vi "VI Tree.vi"   [LabVIEW 2013, in "Fluke 2625A.lvlib"]
doc: "This is the instrument driver for the <INSTRUMENT NAME>. The VI Tree displays all the user-callable VIs of the instrument driver in an organized table."
uses:
  <instrlib>/Fluke 2625A/Fluke 2625A.lvlib
panel:
  # "(c) 2007 <Enter Company Name Here>.  ALL RIGHTS RESERVED."
  # "SEE DIAGRAM\nFOR VI TREE."
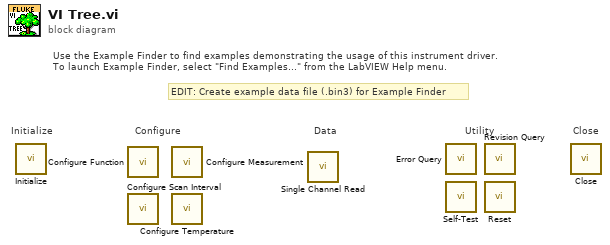
[diagram p0: block diagram]
diagram:
  # "EDIT: Create example data file (.bin3) for Example Finder"
  # "Use the Example Finder to find examples demonstrating the usage of this instrument driver.\nTo launch Example Finder, select \"Find Examples...\" from the LabVIEW Help menu."
  # "Configure"
  # "Utility"
  # "Data"
  # "Close"
  # "Initialize"
  n1 = call <instrlib>:"Initialize.vi"() -> ()  [unwired: 9 in, 3 out]
  n2 = call <instrlib>:"Configure Function.vi"() -> ()  [unwired: 12 in, 4 out]
  n3 = call <instrlib>:"Configure Scan Interval.vi"() -> ()  [unwired: 10 in, 2 out]
  n4 = call <instrlib>:"Configure Measurement.vi"() -> ()  [unwired: 10 in, 2 out]
  n5 = call <instrlib>:"Configure Temperature.vi"() -> ()  [unwired: 9 in, 3 out]
  n6 = call <instrlib>:"Single Channel Read.vi"() -> ()  [unwired: 7 in, 5 out]
  n7 = call <instrlib>:"Error Query.vi"() -> ()  [unwired: 8 in, 4 out]
  n8 = call <instrlib>:"Self-Test.vi"() -> ()  [unwired: 8 in, 4 out]
  n9 = call <instrlib>:"Revision Query.vi"() -> ()  [unwired: 8 in, 4 out]
  n10 = call <instrlib>:"Reset.vi"() -> ()  [unwired: 10 in, 2 out]
  n11 = call <instrlib>:"Close.vi"() -> ()  [unwired: 11 in, 1 out]
